vi "VSG25_Pulse.vi"(0 "Device Handle In":i32, 1 "Run as Subpanel":bool, 2 "Pulse Cluster In":T1 {"Period Factor" items=["Giga", "Mega", "kilo", "Unity", "milli", "micro", "nano", "pico"]; "Width Factor" items=["Giga", "Mega", "kilo", "Unity", "milli", "micro", "nano", "pico"]; "Freq Hz" items=["Hz", "kHz", "MHz", "GHz"]}, 3 "Error In":errorcluster) -> (5 "Device Handle Out":i32, 6 "Pulse Cluster Out":T1 {"Period Factor" items=["Giga", "Mega", "kilo", "Unity", "milli", "micro", "nano", "pico"]; "Width Factor" items=["Giga", "Mega", "kilo", "Unity", "milli", "micro", "nano", "pico"]; "Freq Hz" items=["Hz", "kHz", "MHz", "GHz"]}, 7 "Error Out":errorcluster)   [LabVIEW 2014]
uses:
  Frequency Hertz.ctl
  Factor Control.ctl
  Pulse Cluster.ctl
  sg_lib/VSG25A.lvlib
panel:
  in  "Period Factor":T3 items=["Giga", "Mega", "kilo", "Unity", "milli", "micro", "nano", "pico"]
  in  "Width Factor":T3 items=["Giga", "Mega", "kilo", "Unity", "milli", "micro", "nano", "pico"]
  in  "Stop":bool
  out "Device Selected":bool
  in  "Pulse Period":dbl
  in  "Pulse Width":dbl
  in  "RF On":bool
  in  "Freq Hz":T2 items=["Hz", "kHz", "MHz", "GHz"]
  in  "Amplitude (dBm)":dbl
  in  "Frequency":dbl
  # "Pulse"
  # "(6nS to 25mS)"
  # "(10nS to 1S)"
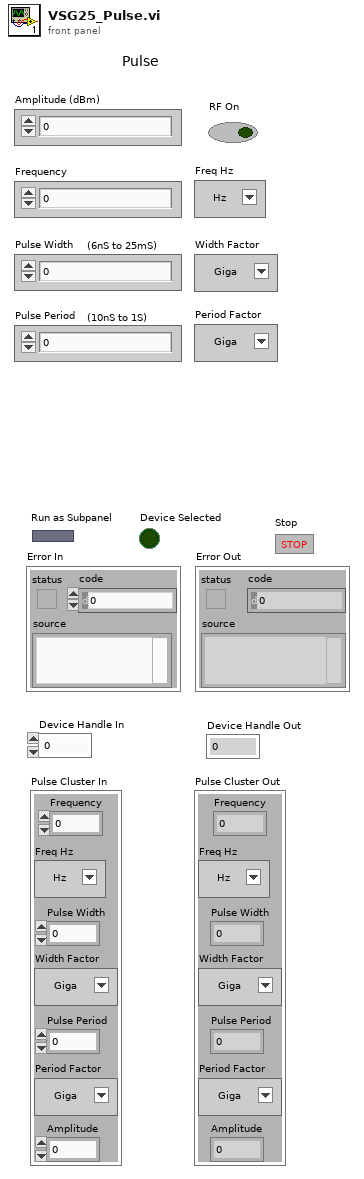
[diagram p1: front panel]
types:
  T1 = typedef "Pulse Cluster.ctl" = cluster{"Frequency":dbl, "Freq Hz":T2, "Pulse Width":dbl, "Amplitude":dbl, "Width Factor":T3, "Pulse Period":dbl, "Period Factor":T3}
  T2 = typedef "Frequency Hertz.ctl" = u16
  T3 = typedef "Factor Control.ctl" = u16
  T4 = enum16{"Init", "Proc Events", "Write VSG25", "Exit"}
  T5 = enum32{"Bad", "Idle", "Run top level", "Running"}
  T6 = enum16{"Check Amplitude ", "Check Frequency", "Check Pulse Width", "Check Pulse Period", "Stop RF", "Set Freq and Amp", "Set Pulse", "Finish"}
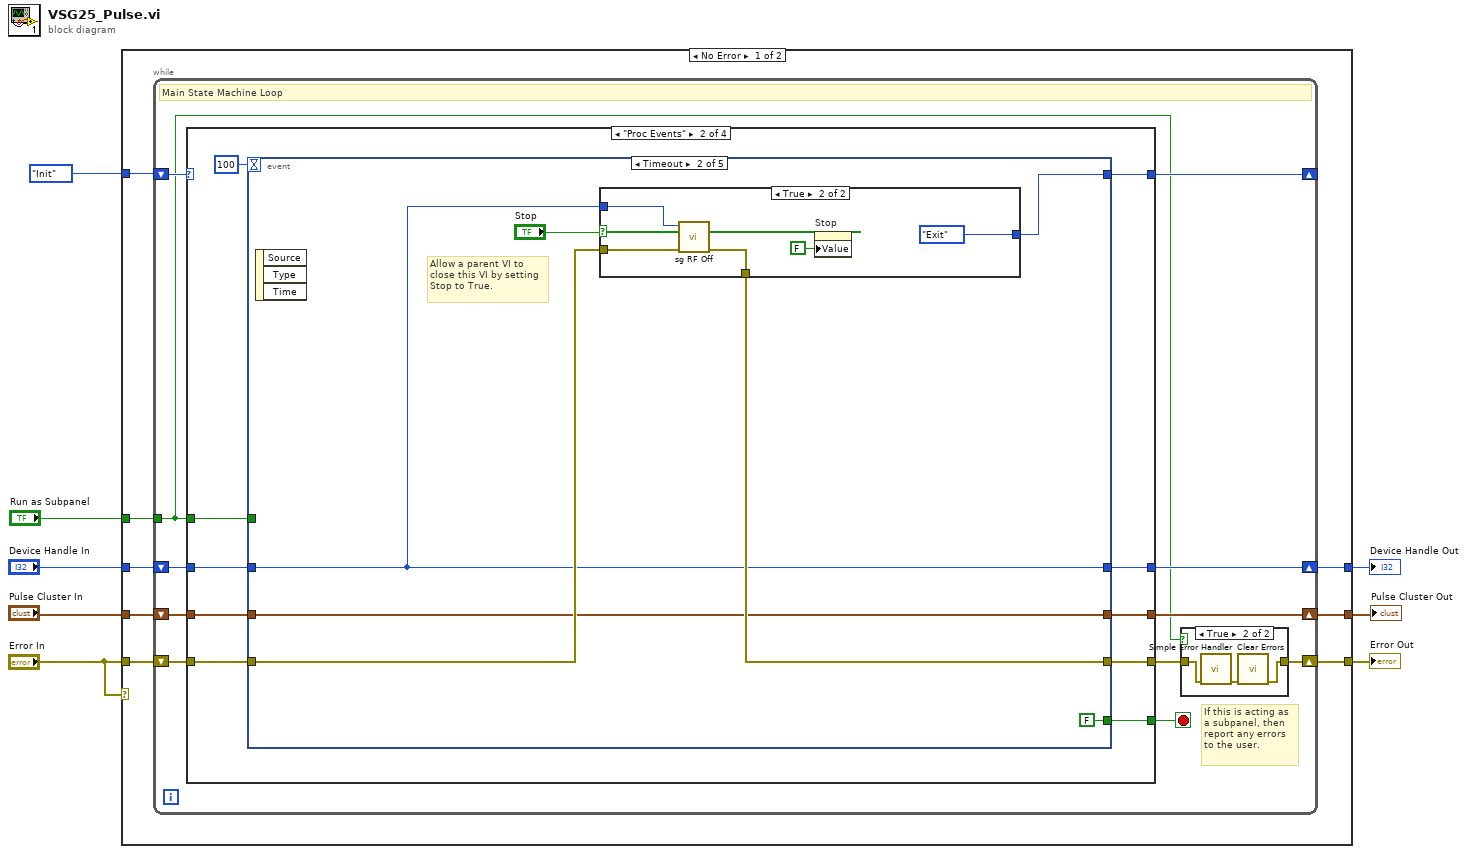
[diagram p0: block diagram]
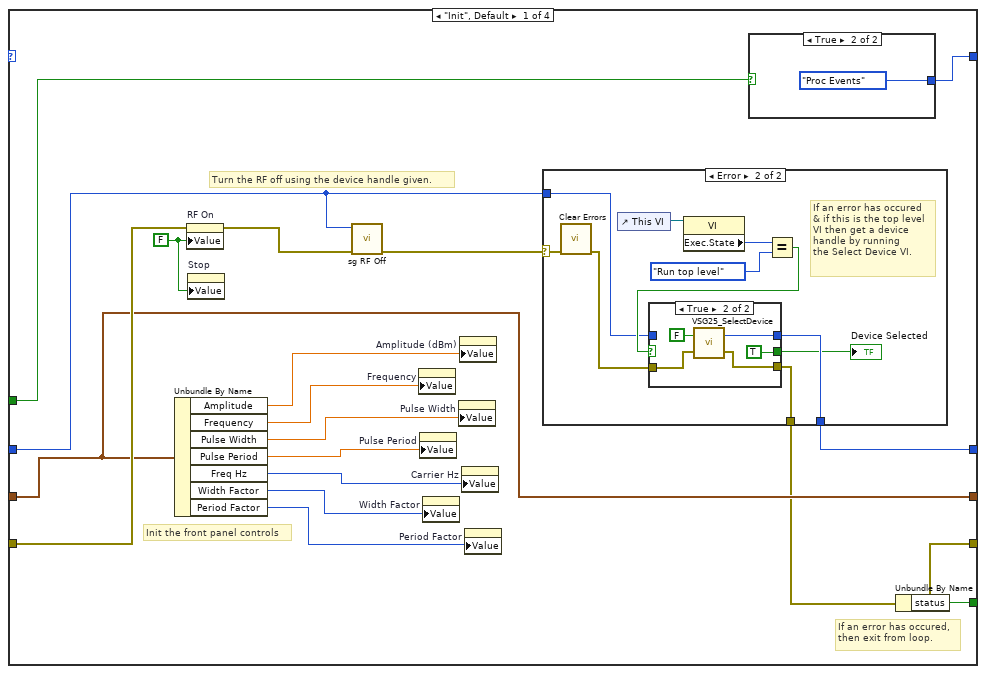
[diagram p3: hidden frame]
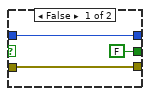
[diagram p5: hidden frame]
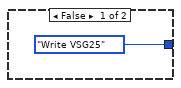
[diagram p6: hidden frame]
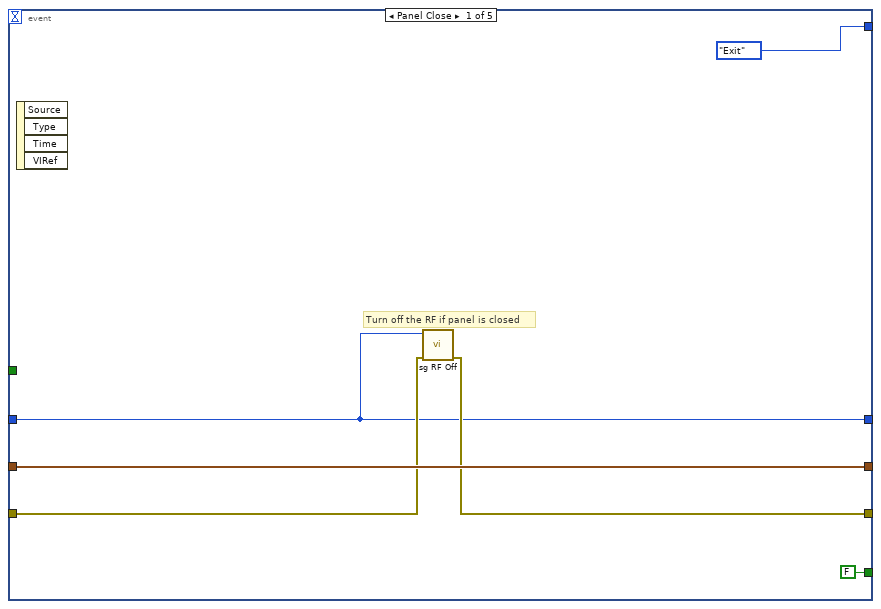
[diagram p7: hidden frame]
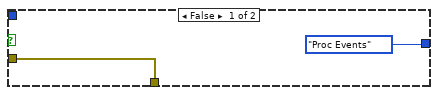
[diagram p8: hidden frame]
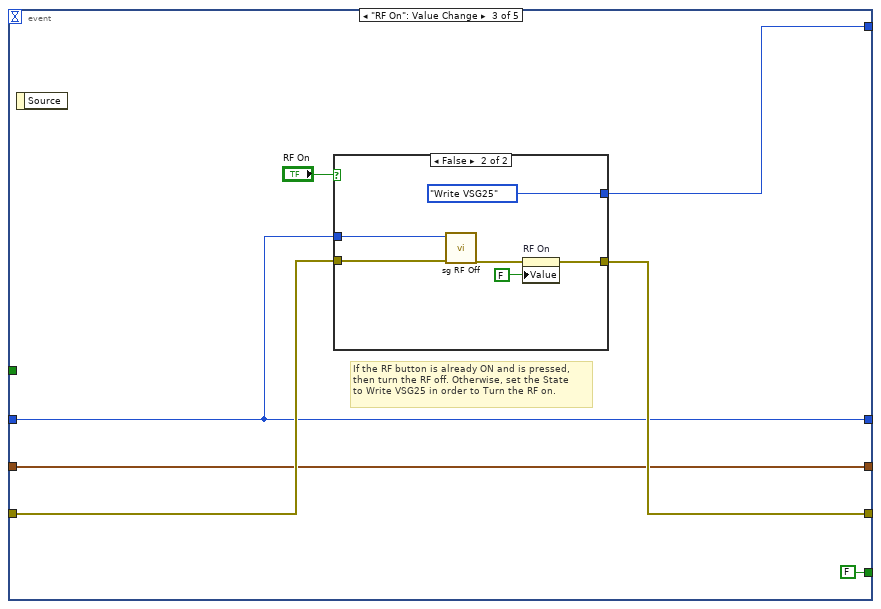
[diagram p9: hidden frame]
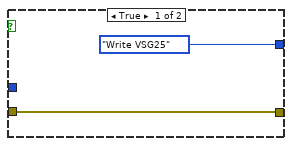
[diagram p10: hidden frame]
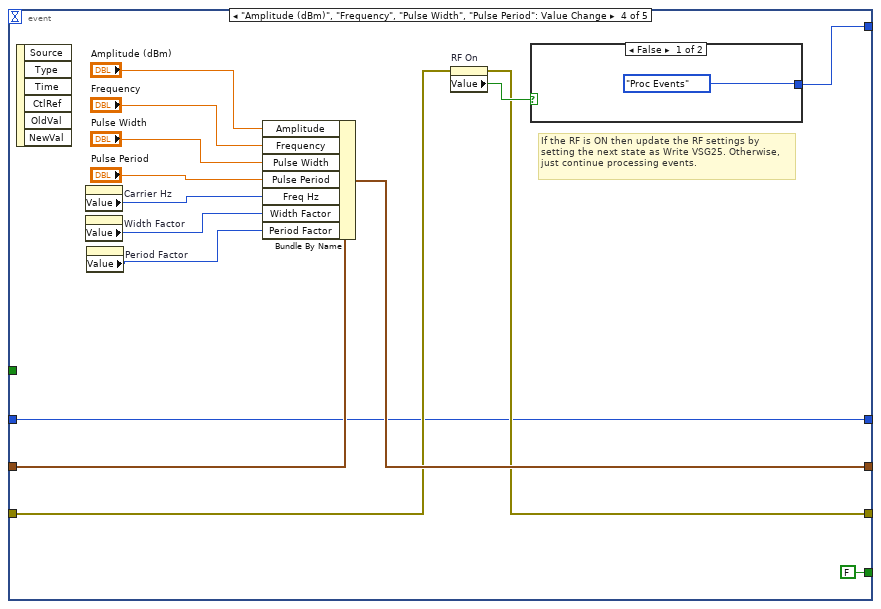
[diagram p11: hidden frame]
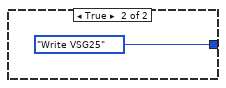
[diagram p12: hidden frame]
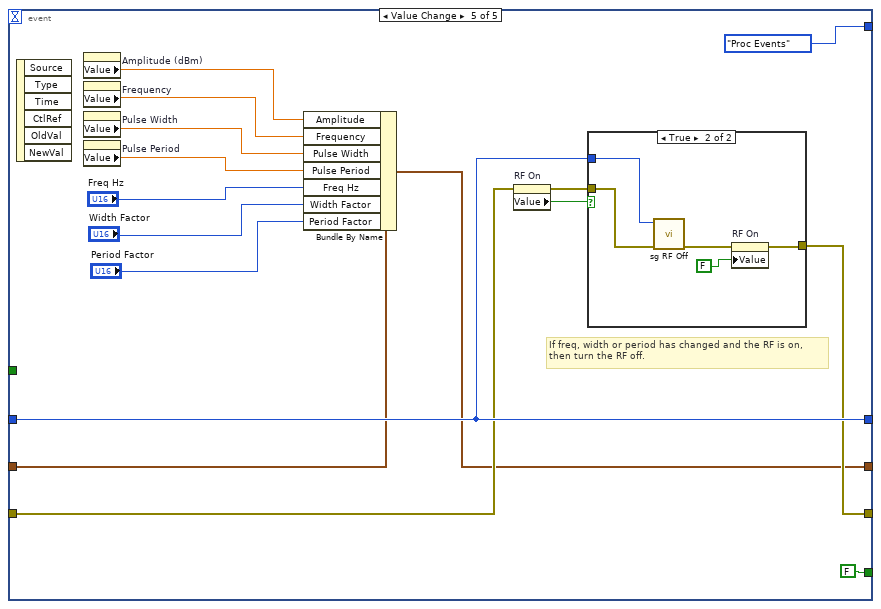
[diagram p13: hidden frame]
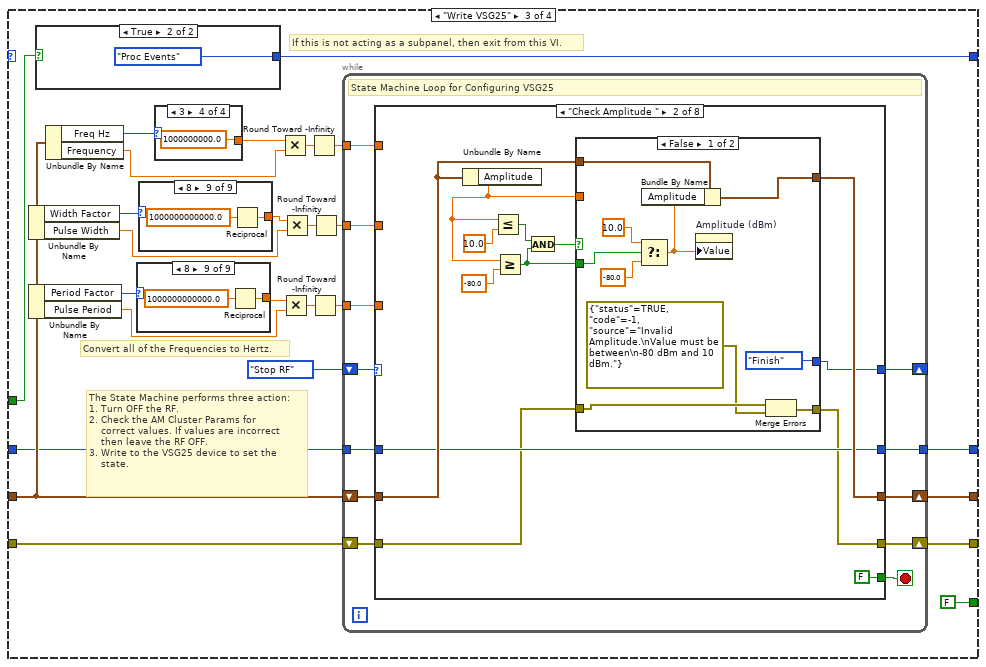
[diagram p15: hidden frame]
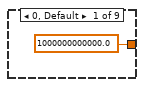
[diagram p16: hidden frame]
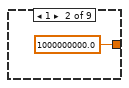
[diagram p17: hidden frame]
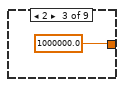
[diagram p18: hidden frame]
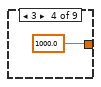
[diagram p19: hidden frame]
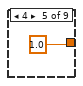
[diagram p20: hidden frame]
diagram:
  n1 = case shown="No Error" "Error In" {
    tunnel: "Error In" -> [w12 w351]
    tunnel: T4."Init" -> [w16 _]
    tunnel: "Run as Subpanel" -> [w15 _]
    tunnel: "Device Handle In" -> [w14 w349]
    tunnel: "Pulse Cluster In" -> [w13 w350]
    tunnel: [w11 w351] -> w4
    tunnel: [w10 w350] -> w1
    tunnel: [w9 w349] -> w3
    frame No Error {
      n2 = while {
        shift-right: [w26] -> _
        shift-left: w16 -> [w27]
        tunnel: w15 -> [w17]
        shift-right: [w18] -> w11
        shift-left: w12 -> [w23]
        shift-right: [w21] -> w10
        shift-left: w13 -> [w24]
        shift-right: [w20] -> w9
        shift-left: w14 -> [w25]
        stop <- w22 stop-if-true
        # "If this is acting as \na subpanel, then\nreport any errors\nto the user."
        # "Main State Machine Loop"
        n3 = case shown="\"Proc Events\"" w27 {
          selector: w27 -> [_ _ _ w344]
          tunnel: [w41 w74 w162 w344] -> w26
          tunnel: w17 -> [w44 w78 w161 _]
          tunnel: w25 -> [w35 w79 w167 w339]
          tunnel: w24 -> [w42 w80 w168 w340]
          tunnel: w23 -> [w43 w81 w172 w341]
          tunnel: [w40 w75 FALSE TRUE] -> w22
          tunnel: [w36 w73 w166 w342] -> w19
          tunnel: [w42 w77 w165 w340] -> w21
          tunnel: [w37 w76 w164 w339] -> w20
          frame "Init", Default {
            w34 = FALSE ("RF On")
            # "Init the front panel controls"
            # "Turn the RF off using the device handle given."
            # "If an error has occured,\nthen exit from loop."
            n4 = Unbundle By Name(w42) -> ("Amplitude"=w49:dbl, "Frequency"=w48:dbl, "Pulse Width"=w47:dbl, "Pulse Period"=w46:dbl, "Freq Hz"=w45:T2, "Width Factor"=w32:T3, "Period Factor"=w33:T3)
            n5 = property on="RF On" class="Bool (strict)"(error in=w43, "Value"=w34) -> (error out=w39:errorcluster)  [unwired: 1 in, 1 out]
            n6 = property on="Stop" class="Bool (strict)"("Value"=w34) -> ()  [unwired: 2 in, 2 out]
            n7 = call "sg RF Off.vi"("error in (no error)"=w39, "device"=w35) -> ("error out"=w38:errorcluster)  [unwired: 8 in, 1 out]
            n8 = property on="Frequency" class="DigNum (strict)"("Value"=w48) -> ()  [unwired: 2 in, 2 out]
            n9 = property on="Pulse Period" class="DigNum (strict)"("Value"=w46) -> ()  [unwired: 2 in, 2 out]
            n10 = property on="Width Factor" class="Ring (strict)"("Value"=w32) -> ()  [unwired: 2 in, 2 out]
            n11 = property on="Pulse Width" class="DigNum (strict)"("Value"=w47) -> ()  [unwired: 2 in, 2 out]
            n12 = property on="Amplitude (dBm)" class="DigNum (strict)"("Value"=w49) -> ()  [unwired: 2 in, 2 out]
            n13 = property on="Carrier Hz" class="Ring (strict)"("Value"=w45) -> ()  [unwired: 2 in, 2 out]
            n14 = property on="Period Factor" class="Ring (strict)"("Value"=w33) -> ()  [unwired: 2 in, 2 out]
            n15 = case shown="Error" w38 {
              selector: w38 -> [w50 w57]
              tunnel: [w51 w55] -> w37
              tunnel: [w50 w54] -> w36
              tunnel: w35 -> [w51 w53]
              frame No Error {
              }
              frame Error {
                # "If an error has occured\n& if this is the top level\nVI then get a device\nhandle by running \nthe Select Device VI."
                n16 = call <vilib>:"Clear Errors.vi"("error in (no error)"=w57) -> ("error out"=w56:errorcluster)  [unwired: 5 in, 1 out]
                n17 = control-ref of="This VI"() -> (w61:refnum<vi>)
                n18 = property class="VI"(reference=w61) -> ("Exec.State"=w60:T5)  [unwired: 1 in, 2 out]
                n19 = Equal?(x=w60, y=T5."Run top level" ("Execution:State 2")) -> (x = y?=w58:bool)
                n20 = case shown="True" w58 {
                  tunnel: [w64 w69] -> w55
                  tunnel: w53 -> [w64 _]
                  tunnel: w56 -> [w63 w67]
                  tunnel: [w63 w66] -> w54
                  tunnel: [FALSE TRUE] -> w52
                  frame False {
                  }
                  frame True {
                    n21 = call "VSG25_SelectDevice.vi"("ErrorIn"=w67, "AutoSel"=FALSE) -> ("ErrorOut"=w66:errorcluster, "deviceHandle"=w69:i32)
                  }
                }
                "Device Selected" <- w52
              }
            }
            n22 = case shown="True" w44 {
              tunnel: [T4."Write VSG25" T4."Proc Events"] -> w41
              frame False {
              }
              frame True {
              }
            }
            n23 = Unbundle By Name(w36) -> ("status"=w40:bool)
          }
          frame "Proc Events" {
            n24 = event shown="[1] Timeout" {
              selector: _ -> [_ _ _ _ _]
              dyn-events: _ -> [_ _ _ _ _]
              timeout: 100 -> [_ _ _ _ _]
              tunnel: w81 -> [w84 w91 w107 w122 w145]
              tunnel: w80 -> [w85 w89 w105 w131 w144]
              tunnel: w79 -> [w82 w88 w104 w120 w147]
              tunnel: w78 -> [_ _ _ _ _]
              tunnel: [w83 w90 w106 w121 w146] -> w73
              tunnel: [w85 w89 w105 w130 w143] -> w77
              tunnel: [w82 w88 w104 w120 w147] -> w76
              tunnel: [FALSE FALSE FALSE FALSE FALSE] -> w75
              tunnel: [T4."Exit" w92 w103 w123 T4."Proc Events"] -> w74
              event Panel Close {
                # "Turn off the RF if panel is closed"
                n25 = event-data() -> ()  [unwired: 1 in, 4 out]
                n26 = call "sg RF Off.vi"("error in (no error)"=w84, "device"=w82) -> ("error out"=w83:errorcluster)  [unwired: 8 in, 1 out]
              }
              event Timeout {
                # "Allow a parent VI to \nclose this VI by setting\nStop to True."
                n27 = event-data() -> ()  [unwired: 1 in, 3 out]
                n28 = case shown="True" "Stop" {
                  tunnel: [T4."Proc Events" T4."Exit"] -> w92
                  tunnel: w91 -> [w95 w100]
                  tunnel: [w95 w99] -> w90
                  tunnel: w88 -> [_ w98]
                  frame False {
                  }
                  frame True {
                    n29 = call "sg RF Off.vi"("error in (no error)"=w100, "device"=w98) -> ("error out"=w99:errorcluster)  [unwired: 8 in, 1 out]
                    n30 = property on="Stop" class="Bool (strict)"("Value"=FALSE ("Stop")) -> ()  [unwired: 2 in, 2 out]
                  }
                }
              }
              event "RF On": Value Change {
                # "If the RF button is already ON and is pressed, \nthen turn the RF off. Otherwise, set the State\nto Write VSG25 in order to Turn the RF on."
                n31 = event-data() -> ()  [unwired: 1 in, 1 out]
                n32 = case shown="False" "RF On" {
                  tunnel: [w109 w114] -> w106
                  tunnel: w107 -> [w109 w116]
                  tunnel: w104 -> [_ w115]
                  tunnel: [T4."Write VSG25" T4."Write VSG25"] -> w103
                  frame True {
                  }
                  frame False {
                    n33 = call "sg RF Off.vi"("error in (no error)"=w116, "device"=w115) -> ("error out"=w113:errorcluster)  [unwired: 8 in, 1 out]
                    n34 = property on="RF On" class="Bool (strict)"(error in=w113, "Value"=FALSE ("RF On")) -> (error out=w114:errorcluster)  [unwired: 1 in, 1 out]
                  }
                }
              }
              event "Amplitude (dBm)", "Frequency", "Pulse Width", "Pulse Period": Value Change {
                # "If the RF is ON then update the RF settings by\nsetting the next state as Write VSG25. Otherwise,\njust continue processing events."
                n35 = event-data() -> ()  [unwired: 1 in, 6 out]
                n36 = property on="Carrier Hz" class="Ring (strict)"() -> ("Value"=w125:T2)  [unwired: 2 in, 2 out]
                n37 = property on="Width Factor" class="Ring (strict)"() -> ("Value"=w118:T3)  [unwired: 2 in, 2 out]
                n38 = property on="Period Factor" class="Ring (strict)"() -> ("Value"=w117:T3)  [unwired: 2 in, 2 out]
                n39 = Bundle By Name(cluster=w131, "Amplitude"="Amplitude (dBm)", "Frequency"="Frequency", "Pulse Width"="Pulse Width", "Pulse Period"="Pulse Period", "Freq Hz"=w125, "Width Factor"=w118, "Period Factor"=w117) -> (w130:T1)
                n40 = property on="RF On" class="Bool (strict)"(error in=w122) -> (error out=w121:errorcluster, "Value"=w124:bool)  [unwired: 1 in, 1 out]
                n41 = case shown="False" w124 {
                  tunnel: [T4."Proc Events" T4."Write VSG25"] -> w123
                  frame False {
                  }
                  frame True {
                  }
                }
              }
              event Value Change {
                # "If freq, width or period has changed and the RF is on,\nthen turn the RF off."
                n42 = event-data() -> ()  [unwired: 1 in, 6 out]
                n43 = property on="Amplitude (dBm)" class="DigNum (strict)"() -> ("Value"=w142:dbl)  [unwired: 2 in, 2 out]
                n44 = property on="Frequency" class="DigNum (strict)"() -> ("Value"=w141:dbl)  [unwired: 2 in, 2 out]
                n45 = property on="Pulse Width" class="DigNum (strict)"() -> ("Value"=w140:dbl)  [unwired: 2 in, 2 out]
                n46 = property on="Pulse Period" class="DigNum (strict)"() -> ("Value"=w139:dbl)  [unwired: 2 in, 2 out]
                n47 = Bundle By Name(cluster=w144, "Amplitude"=w142, "Frequency"=w141, "Pulse Width"=w140, "Pulse Period"=w139, "Freq Hz"="Freq Hz", "Width Factor"="Width Factor", "Period Factor"="Period Factor") -> (w143:T1)
                n48 = property on="RF On" class="Bool (strict)"(error in=w145) -> (error out=w149:errorcluster, "Value"=w148:bool)  [unwired: 1 in, 1 out]
                n49 = case shown="True" w148 {
                  tunnel: [w150 w151] -> w146
                  tunnel: w149 -> [w150 w155]
                  tunnel: w147 -> [_ w154]
                  frame False {
                  }
                  frame True {
                    n50 = call "sg RF Off.vi"("error in (no error)"=w155, "device"=w154) -> ("error out"=w152:errorcluster)  [unwired: 8 in, 1 out]
                    n51 = property on="RF On" class="Bool (strict)"(error in=w152, "Value"=FALSE ("RF On")) -> (error out=w151:errorcluster)  [unwired: 1 in, 1 out]
                  }
                }
              }
            }
          }
          frame "Write VSG25" {
            # "If this is not acting as a subpanel, then exit from this VI."
            # "Convert all of the Frequencies to Hertz."
            # "The State Machine performs three action:\n1. Turn OFF the RF.\n2. Check the AM Cluster Params for \n    correct values. If values are incorrect\n    then leave the RF OFF.\n3. Write to the VSG25 device to set the\n    state."
            n52 = Unbundle By Name(w168) -> ("Width Factor"=w160:T3, "Pulse Width"=w176:dbl)
            n53 = Unbundle By Name(w168) -> ("Period Factor"=w157:T3, "Pulse Period"=w174:dbl)
            n54 = case shown="True" w161 {
              tunnel: [T4."Exit" T4."Proc Events"] -> w162
              frame False {
              }
              frame True {
              }
            }
            n55 = Unbundle By Name(w168) -> ("Freq Hz"=w179:T2, "Frequency"=w177:dbl)
            n56 = case shown="8" w157 {
              tunnel: [1000000000000.0 1000000000.0 ("y") 1000000.0 ("y") 1000.0 ("y") 1.0 ("y") w187 w189 w191 w193] -> w158
              frame 0, Default {
              }
              frame 1 {
              }
              frame 2 {
              }
              frame 3 {
              }
              frame 4 {
              }
              frame 5 {
                n57 = Reciprocal(x=1000.0 ("y")) -> (1/x=w187:dbl)
              }
              frame 6 {
                n58 = Reciprocal(x=1000000.0 ("y")) -> (1/x=w189:dbl)
              }
              frame 7 {
                n59 = Reciprocal(x=1000000000.0 ("y")) -> (1/x=w191:dbl)
              }
              frame 8 {
                n60 = Reciprocal(x=1000000000000.0) -> (1/x=w193:dbl)
              }
            }
            n61 = case shown="8" w160 {
              tunnel: [1000000000000.0 1000000000.0 ("y") 1000000.0 ("y") 1000.0 ("y") 1.0 ("y") w200 w202 w204 w206] -> w159
              frame 0, Default {
              }
              frame 1 {
              }
              frame 2 {
              }
              frame 3 {
              }
              frame 4 {
              }
              frame 5 {
                n62 = Reciprocal(x=1000.0 ("y")) -> (1/x=w200:dbl)
              }
              frame 6 {
                n63 = Reciprocal(x=1000000.0 ("y")) -> (1/x=w202:dbl)
              }
              frame 7 {
                n64 = Reciprocal(x=1000000000.0 ("y")) -> (1/x=w204:dbl)
              }
              frame 8 {
                n65 = Reciprocal(x=1000000000000.0) -> (1/x=w206:dbl)
              }
            }
            n66 = case shown="3" w179 {
              tunnel: [1.0 ("y") 1000.0 ("y") 1000000.0 ("y") 1000000000.0 ("y")] -> w178
              frame 0, Default {
              }
              frame 1 {
              }
              frame 2 {
              }
              frame 3 {
              }
            }
            n67 = Multiply(x=w178, y=w177) -> (x*y=w180:dbl)
            n68 = Multiply(x=w158, y=w174) -> (x*y=w173:dbl)
            n69 = Multiply(x=w159, y=w176) -> (x*y=w175:dbl)
            n70 = Round Toward -Infinity(1:w180) -> (0:w171:dbl)
            n71 = Round Toward -Infinity(1:w173) -> (0:w169:dbl)
            n72 = Round Toward -Infinity(1:w175) -> (0:w170:dbl)
            n73 = while {
              tunnel: w171 -> [w219]
              tunnel: w170 -> [w218]
              tunnel: w169 -> [w217]
              tunnel: w167 -> [w215]
              tunnel: [w212] -> w164
              shift-right: [w214] -> w166
              shift-left: w172 -> [w220]
              shift-right: [w213] -> w165
              shift-left: w168 -> [w216]
              shift-right: [w209] -> _
              shift-left: T6."Stop RF" -> [w210]
              stop <- w211 stop-if-true
              # "State Machine Loop for Configuring VSG25"
              n74 = case shown="\"Check Amplitude \"" w210 {
                selector: w210 -> [_ _ _ _ _ _ _ w326]
                tunnel: w220 -> [w226 w229 w258 w276 w294 w315 w322 w327]
                tunnel: w219 -> [_ _ w263 _ _ w313 _ _]
                tunnel: w218 -> [_ _ _ w280 _ _ w320 _]
                tunnel: w217 -> [_ _ _ _ w298 _ w319 _]
                tunnel: w216 -> [w224 w233 w259 w278 w296 w316 w325 w328]
                tunnel: w215 -> [w223 w231 w260 w277 w295 w312 w318 w329]
                tunnel: [w225 w228 w257 w275 w293 w314 w321 w327] -> w214
                tunnel: [w224 w232 w259 w278 w296 w316 w325 w328] -> w213
                tunnel: [w223 w231 w260 w277 w295 w312 w318 w329] -> w212
                tunnel: [FALSE FALSE FALSE FALSE FALSE FALSE FALSE TRUE] -> w211
                tunnel: [T6."Check Amplitude " w227 w256 w274 w292 T6."Set Pulse" T6."Finish" w326] -> w209
                frame "Stop RF", Default {
                  n75 = call "sg RF Off.vi"("error in (no error)"=w226, "device"=w223) -> ("error out"=w225:errorcluster)  [unwired: 8 in, 1 out]
                }
                frame "Check Amplitude " {
                  n76 = Unbundle By Name(w233) -> ("Amplitude"=w239:dbl)
                  n77 = Less Or Equal?(x=w239, y=10.0) -> (x <= y?=w235:bool)
                  n78 = Greater Or Equal?(x=w239, y=-80.0) -> (x >= y?=w238:bool)
                  n79 = And(x=w235, y=w238) -> (x .and. y?=w234:bool)
                  n80 = case shown="False" w234 {
                    tunnel: w238 -> [w249 _]
                    tunnel: w239 -> [_ w254]
                    tunnel: w233 -> [w246 w253]
                    tunnel: [w245 w252] -> w232
                    tunnel: [T6."Finish" T6."Check Frequency"] -> w227
                    tunnel: w229 -> [w243 w251]
                    tunnel: [w241 w251] -> w228
                    frame False {
                      n81 = Select(t=10.0, s=w249, f=-80.0) -> (s? t:f=w244:dbl)
                      n82 = Bundle By Name(cluster=w246, "Amplitude"=w244) -> (w245:T1)
                      n83 = property on="Amplitude (dBm)" class="DigNum (strict)"("Value"=w244) -> ()  [unwired: 2 in, 2 out]
                      n84 = Merge Errors(w243, errorcluster {"status"=TRUE, "code"=-1, "source"="Invalid Amplitude.\nValue must be between\n-80 dBm and 10 dBm."} ("error constant")) -> (w241:errorcluster)
                    }
                    frame True {
                      n85 = Round Toward -Infinity(1:w254) -> (0:w255:dbl)
                      n86 = Bundle By Name(cluster=w253, "Amplitude"=w255) -> (w252:T1)
                    }
                  }
                }
                frame "Check Frequency" {
                  n87 = Greater Or Equal?(x=w263, y=80000000.0) -> (x >= y?=w267:bool)
                  n88 = Less Or Equal?(x=w263, y=2500000000.0) -> (x <= y?=w262:bool)
                  n89 = Compound Arithmetic op=AND(w267, w262) -> (w266:bool)
                  n90 = case shown="True" w266 {
                    tunnel: [T6."Finish" T6."Check Pulse Width"] -> w256
                    tunnel: w258 -> [w270 w273]
                    tunnel: [w271 w273] -> w257
                    frame False {
                      n91 = Merge Errors(w270, errorcluster {"status"=TRUE, "code"=-1, "source"="Carrier frequency must \nbe greater than 80 MHz\nand less than 2.5 GHz."} ("error constant")) -> (w271:errorcluster)
                    }
                    frame True {
                    }
                  }
                }
                frame "Check Pulse Width" {
                  n92 = Greater Or Equal?(x=w280, y=6e-09) -> (x >= y?=w285:bool)
                  n93 = Less Or Equal?(x=w280, y=0.025) -> (x <= y?=w281:bool)
                  n94 = Compound Arithmetic op=AND(w285, w281) -> (w284:bool)
                  n95 = case shown="True" w284 {
                    tunnel: [T6."Finish" T6."Check Pulse Period"] -> w274
                    tunnel: w276 -> [w289 w291]
                    tunnel: [w287 w291] -> w275
                    frame False {
                      n96 = Merge Errors(w289, errorcluster {"status"=TRUE, "code"=-1, "source"="Pulse Width must \nbe greater than 6nS\nand less than 25mS."} ("error constant")) -> (w287:errorcluster)
                    }
                    frame True {
                    }
                  }
                }
                frame "Check Pulse Period" {
                  n97 = Greater Or Equal?(x=w298, y=1e-08) -> (x >= y?=w303:bool)
                  n98 = Less Or Equal?(x=w298, y=1.0) -> (x <= y?=w299:bool)
                  n99 = Compound Arithmetic op=AND(w303, w299) -> (w302:bool)
                  n100 = case shown="False" w302 {
                    tunnel: [T6."Finish" T6."Set Freq and Amp"] -> w292
                    tunnel: w294 -> [w306 w309]
                    tunnel: [w307 w309] -> w293
                    frame False {
                      n101 = Merge Errors(w306, errorcluster {"status"=TRUE, "code"=-1, "source"="Pulse Period must \nbe greater than 10nS\nand less than 1 second."} ("error constant")) -> (w307:errorcluster)
                    }
                    frame True {
                    }
                  }
                }
                frame "Set Freq and Amp" {
                  n102 = Unbundle By Name(w316) -> ("Amplitude"=w317:dbl)
                  n103 = call "sg Set Frequency Amplitude.vi"("error in (no error)"=w315, "amplitude"=w317, "frequency"=w313, "device"=w312) -> ("error out"=w314:errorcluster)  [unwired: 6 in, 1 out]
                }
                frame "Set Pulse" {
                  n104 = call "sg Set Pulse.vi"("error in (no error)"=w322, "width"=w320, "period"=w319, "device"=w318) -> ("error out"=w321:errorcluster)  [unwired: 6 in, 1 out]
                }
                frame "Finish" {
                  # "If no errors have occured, then indicate that the RF is ON."
                  n105 = case shown="Error" w327 {
                    tunnel: [TRUE FALSE] -> w331
                    frame No Error {
                    }
                    frame Error {
                    }
                  }
                  n106 = property on="RF On" class="Bool (strict)"("Value"=w331) -> ()  [unwired: 2 in, 2 out]
                }
              }
            }
          }
          frame "Exit" {
            # "If a device handle was\nacquired using the \nSelect Device VI, then\nclose the handle \nbefore exiting."
            n107 = local read "Device Selected"() -> (w338:bool)
            n108 = case shown="True" w338 {
              tunnel: w339 -> [_ w348]
              tunnel: w341 -> [w345 w347]
              tunnel: [w345 w346] -> w342
              frame False {
              }
              frame True {
                n109 = call "sg Close Device.vi"("error in (no error)"=w347, "device"=w348) -> ("error out"=w346:errorcluster)  [unwired: 8 in, 1 out]
              }
            }
          }
        }
        n110 = case shown="True" w17 {
          tunnel: w19 -> [w28 w30]
          tunnel: [w28 w31] -> w18
          frame False {
          }
          frame True {
            n111 = call <vilib>:"Simple Error Handler.vi"("error in (no error)"=w30) -> ("error out"=w29:errorcluster)  [unwired: 4 in, 4 out]
            n112 = call <vilib>:"Clear Errors.vi"("error in (no error)"=w29) -> ("error out"=w31:errorcluster)  [unwired: 5 in, 1 out]
          }
        }
      }
    }
    frame Error {
    }
  }
  "Error Out" <- w4
  "Device Handle Out" <- w3
  "Pulse Cluster Out" <- w1
